vi "virtual generation.vi"() -> ()   [LabVIEW 2023]
uses:
  <vilib>/measure/NI_MABase.lvlib
panel:
  in  "stop":bool
  out "Waveform Chart":waveform(dbl)(graph)
  in  "square wave duty":dbl(knob) scale=0.0..100.0
  in  "frequency":dbl(knob) scale=0.0..10.0
  in  "amplitude":dbl(knob) scale=0.0..10.0
  in  "DC offset":dbl(knob) scale=-5.0..5.0
  in  "signal type":T1(ring)
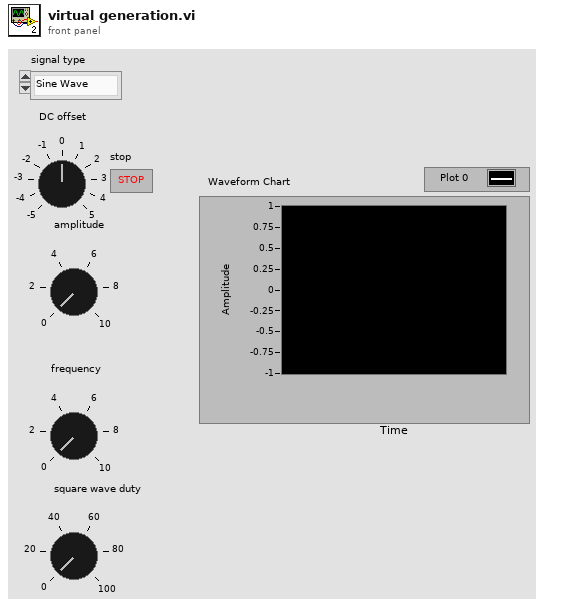
[diagram p1: front panel]
types:
  T1 = enum16{"Sine Wave", "Triangle Wave", "Square Wave", "Sawtooth Wave"}
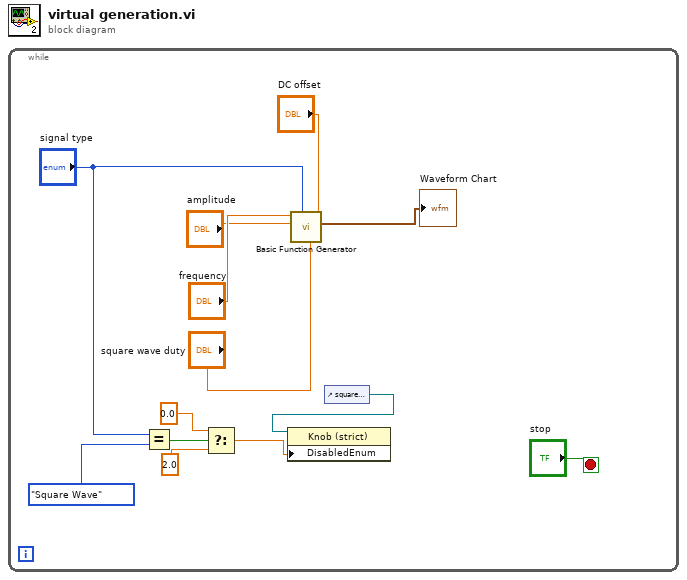
[diagram p0: block diagram]
diagram:
  n1 = while {
    stop <- "stop" stop-if-true
    n2 = Equal?(x="signal type", y=T1."Square Wave") -> (x = y?=w5:bool)
    n3 = Select(t=0.0, s=w5, f=2.0) -> (s? t:f=w1:dbl)
    n4 = call <vilib>:"Basic Function Generator.vi"("offset"="DC offset", "square wave duty cycle (%)"="square wave duty", "signal type"="signal type", "amplitude"="amplitude", "frequency"="frequency") -> ("signal out"=→"Waveform Chart":waveform(dbl))  [unwired: 4 in, 2 out]
    n5 = control-ref of="square wave duty"() -> (w2:refnum<vi>)
    n6 = property class="Knob (strict)"(reference=w2, "DisabledEnum"=w1) -> ()  [unwired: 1 in, 2 out]
  }
